vi "uMsg Update Timestamp.vi"(8 "error in (no error)":errorcluster, 10 "Timestamp":u32, 11 "uMsg in":refnum<class "uMsg.lvclass">) -> (0 "error out":errorcluster, 3 "uMsg out":refnum<class "uMsg.lvclass">)   [LabVIEW 2021, in "uFramework.lvlib" / "uMsg.lvclass"]
doc: "If the message is not timestamped in itself and a value is not provided to the timestamp teminal on the connector pane, then the method automatically applies the current tick count as time stamp.\n\nIf a timestamp is wired to the copane, the timestamp in the uMsg is overwritten.\n\nSimply wire in a zero to the input terminal in order to attach a timestamp if one does not exist.\n\nThe method does not execute on an error in."
uses:
  uMsg.lvclass
  uMsg.lvclass/uMsg.ctl
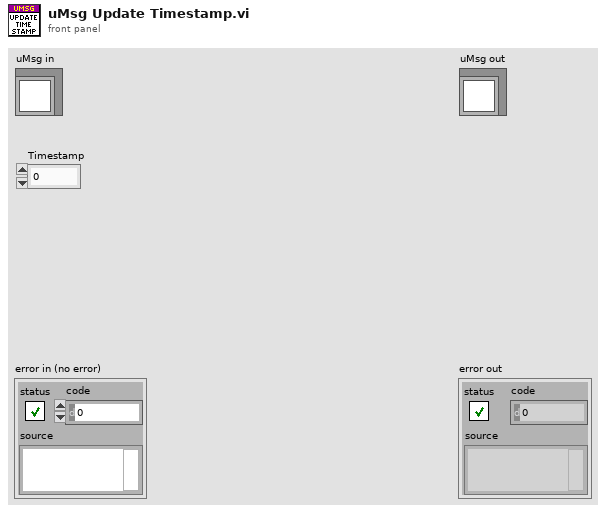
[diagram p1: front panel]
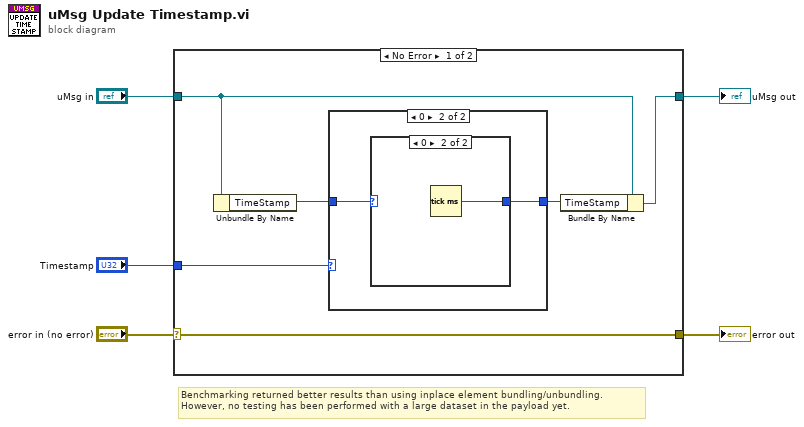
[diagram p0: block diagram]
diagram:
  # "Benchmarking returned better results than using inplace element bundling/unbundling.\nHowever, no testing has been performed with a large dataset in the payload yet."
  n1 = case shown="No Error" "error in (no error)" {
    selector: "error in (no error)" -> [w9 w18]
    tunnel: [w9 w18] -> w5
    tunnel: [w11 w17] -> w4
    tunnel: "uMsg in" -> [w10 w17]
    tunnel: "Timestamp" -> [w8 _]
    frame No Error {
      n2 = Unbundle By Name(w10) -> ("TimeStamp"=w6:u32)
      n3 = case shown="0" w8 {
        selector: w8 -> [w12 _]
        tunnel: [w12 w13] -> w7
        tunnel: w6 -> [_ w14]
        frame Default {
        }
        frame 0 {
          n4 = case shown="0" w14 {
            selector: w14 -> [w15 _]
            tunnel: [w15 w16] -> w13
            frame Default {
            }
            frame 0 {
              n5 = Tick Count (ms)() -> (millisecond timer value=w16:u32)
            }
          }
        }
      }
      n6 = Bundle By Name(cluster=w10, "TimeStamp"=w7) -> (w11:refnum<class "uMsg.lvclass">)
    }
    frame Error {
    }
  }
  "error out" <- w5
  "uMsg out" <- w4
